vi "InitialConditionTest.vi"(0 "VI Reference In":refnum<vi>, 11 "error in":errorcluster) -> (4 "VI Reference Out":refnum<vi>, 15 "error out":errorcluster)   [LabVIEW 2016]
uses:
  Car Wash 16.0/Controls/Wash Options.ctl
  Car Wash 16.0/Controls/Car Wash Indicators.ctl
  main/apis/Assert/AssertControlValueCompare/AssertControlValueEqual.vi
  Car Wash 16.0/Car Wash.lvlib
  <vilib>/addons/_JKI Toolkits/Caraya/classes/Test/Test.lvclass
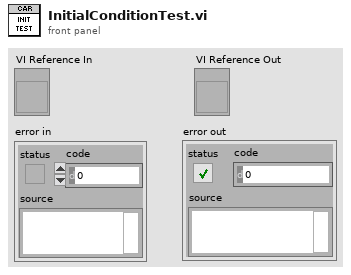
[diagram p1: front panel]
types:
  T1 = typedef "Car Wash.lvlib/Car Wash Indicators.ctl" = cluster{"Underbody Wash":bool, "Bug Remover":bool, "Pre-Soak":bool, "High Pressure Wash":bool, "Low Pressure Wax":bool, "Spot Free Rinse":bool, "Tire Shine Foam":bool, "Air Dry":bool, "Vehicle Out of Position":bool}
  T2 = typedef "Car Wash.lvlib/Wash Options.ctl" = cluster{"Underbody Wash":bool, "Bug Remover":bool, "Pre-Soak":bool, "High Pressure Wash":bool, "Low Pressure Wax":bool, "Spot Free Rinse":bool, "Tire Shine Foam":bool, "Air Dry":bool}
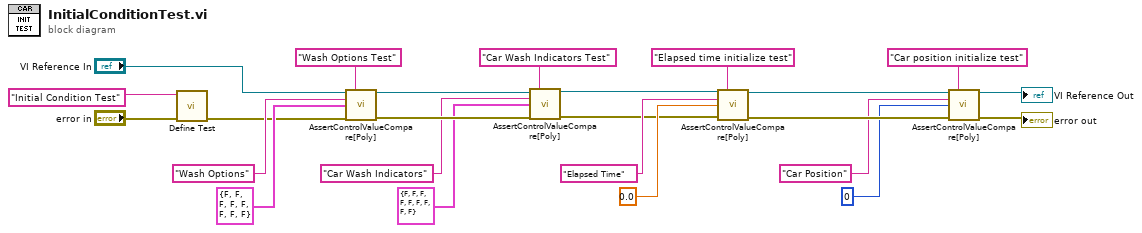
[diagram p0: block diagram]
diagram:
  n1 = call <vilib>:"Define Test.vi"("error in (no error)"="error in", "Label (VI Title)"="Initial Condition Test") -> ("error out"=w2:errorcluster)  [unwired: 9 in]
  n2 = call-poly "AssertControlValueCompare[Poly].vi"("VI Reference In"="VI Reference In", "Label"="Wash Options Test", "Control Name"="Wash Options", "Control Value"=T2 {"Underbody Wash"=FALSE, "Bug Remover"=FALSE, "Pre-Soak"=FALSE, "High Pressure Wash"=FALSE, "Low Pressure Wax"=FALSE, "Spot Free Rinse"=FALSE, "Tire Shine Foam"=FALSE, "Air Dry"=FALSE} ("Wash Options"), "Error In"=w2) -> ("VI Reference Out"=w10:refnum<vi>, "Error Out"=w13:errorcluster)  [unwired: 9 in]
  n3 = call-poly "AssertControlValueCompare[Poly].vi"("VI Reference In"=w10, "Label"="Car Wash Indicators Test", "Control Name"="Car Wash Indicators", "Control Value"=T1 {"Underbody Wash"=FALSE, "Bug Remover"=FALSE, "Pre-Soak"=FALSE, "High Pressure Wash"=FALSE, "Low Pressure Wax"=FALSE, "Spot Free Rinse"=FALSE, "Tire Shine Foam"=FALSE, "Air Dry"=FALSE, "Vehicle Out of Position"=FALSE} ("Car Wash Indicators"), "Error In"=w13) -> ("VI Reference Out"=w11:refnum<vi>, "Error Out"=w12:errorcluster)  [unwired: 9 in]
  n4 = call-poly "AssertControlValueCompare[Poly].vi"("VI Reference In"=w11, "Label"="Elapsed time initialize test", "Control Name"="Elapsed Time", "Control Value"=0.0, "Error In"=w12) -> ("VI Reference Out"=w19:refnum<vi>, "Error Out"=w20:errorcluster)  [unwired: 9 in]
  n5 = call-poly "AssertControlValueCompare[Poly].vi"("VI Reference In"=w19, "Label"="Car position initialize test", "Control Name"="Car Position", "Control Value"=u8 0, "Error In"=w20) -> ("VI Reference Out"=→"VI Reference Out":refnum<vi>, "Error Out"=→"error out":errorcluster)  [unwired: 9 in]
